vi "Variable Operation.vi"(8 "error in (no error)":errorcluster, 9 "Variable Tree":refnum<vi>, 10 "Variable Data":T1, 11 "Project in":refnum<class "Project.lvclass">) -> (0 "error out":errorcluster, 1 "Successful":bool, 3 "Project out":refnum<class "Project.lvclass">)   [LabVIEW 2015, in "Project.lvclass"]
uses:
  Project.lvclass
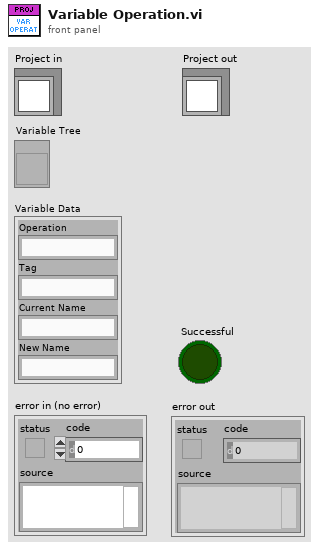
[diagram p1: front panel]
types:
  T1 = cluster{"Operation":string, "Tag":string, "Current Name":string, "New Name":string}
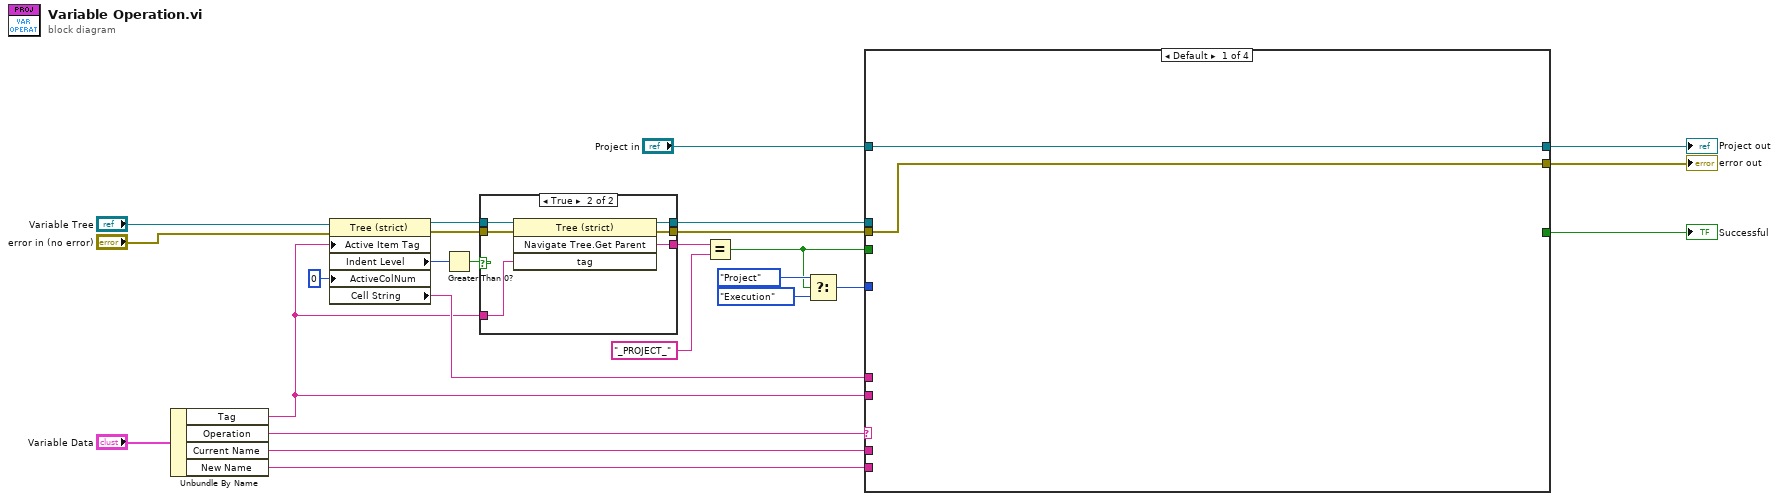
[diagram p0: block diagram]
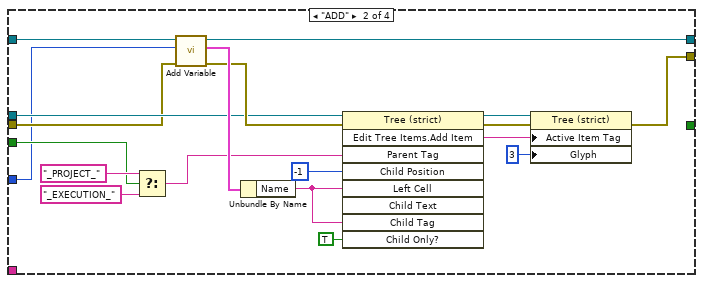
[diagram p2: hidden frame]
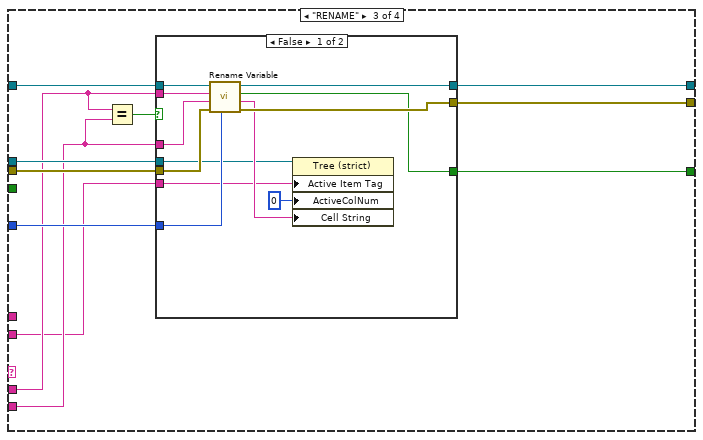
[diagram p3: hidden frame]
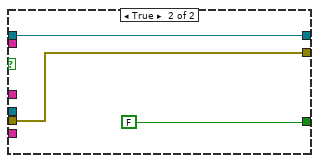
[diagram p4: hidden frame]
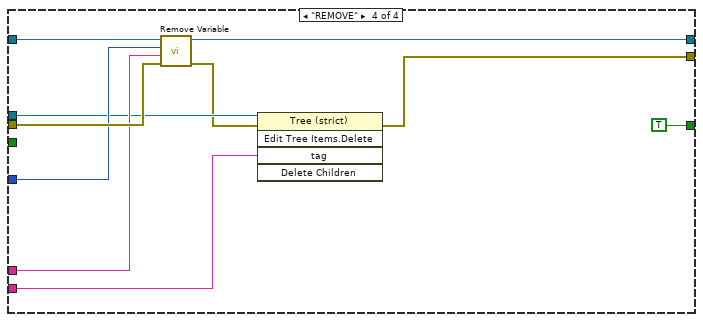
[diagram p5: hidden frame]
diagram:
  n1 = Unbundle By Name("Variable Data") -> ("Tag"=w4:string, "Operation"=w3:string, "Current Name"=w2:string, "New Name"=w1:string)
  n2 = property class="Tree (strict)"(reference="Variable Tree", error in="error in (no error)", "Active Item Tag"=w4, "ActiveColNum"=0 ("Active Cell:Active Column Number")) -> (reference out=w20:refnum<vi>, error out=w19:errorcluster, "Indent Level"=w15:i32, "Cell String"=w13:string)
  n3 = Greater Than 0?(x=w15) -> (x > 0?=w21:bool)
  n4 = case shown="True" w21 {
    tunnel: w4 -> [w28 w34]
    tunnel: w20 -> [w26 w33]
    tunnel: w19 -> [w27 w32]
    tunnel: [w28 w31] -> w18
    tunnel: [w26 w30] -> w17
    tunnel: [w27 w29] -> w16
    frame False {
    }
    frame True {
      n5 = invoke class="Tree (strict)" method="Navigate Tree.Get Parent"(reference=w33, error in=w32, "tag"=w34) -> (reference out=w30:refnum<vi>, error out=w29:errorcluster, "Navigate Tree:Get Parent"=w31:string)  [unwired: 1 in, 1 out]
    }
  }
  n6 = Equal?(x=w18, y="_PROJECT_") -> (x = y?=w9:bool)
  n7 = Select(t=enum16{"Project", "Execution"}."Project" ("Variable Type"), s=w9, f=enum16{"Project", "Execution"}."Execution" ("Variable Type")) -> (s? t:f=w8:enum16{"Project", "Execution"})
  n8 = case shown="Default" w3 {
    tunnel: "Project in" -> [w36 w55 w66 w91]
    tunnel: [w36 w51 w65 w90] -> w24
    tunnel: [w35 w45 w63 w83] -> w23
    tunnel: w17 -> [_ w43 w60 w86]
    tunnel: w9 -> [_ w39 _ _]
    tunnel: w16 -> [w35 w38 w64 w89]
    tunnel: w13 -> [_ _ _ w88]
    tunnel: [_ _ w62 TRUE ("Successful")] -> w12
    tunnel: w8 -> [_ w37 w59 w87]
    tunnel: w4 -> [_ _ w56 w84]
    tunnel: w2 -> [_ _ w58 _]
    tunnel: w1 -> [_ _ w57 _]
    frame Default {
    }
    frame "ADD" {
      n9 = Select(t="_PROJECT_", s=w39, f="_EXECUTION_" ("Child Tag")) -> (s? t:f=w40:string)
      n10 = call-dynamic "Add Variable.vi"("error in (no error)"=w38, "Variable Type"=w37, "Project in"=w55) -> ("error out"=w52:errorcluster, "Variable"=w54:cluster{"Name":string, "Value":variant}, "Project out"=w51:refnum<class "Project.lvclass">)  [unwired: 6 in]
      n11 = Unbundle By Name(w54) -> ("Name"=w53:string)
      n12 = invoke class="Tree (strict)" method="Edit Tree Items.Add Item"(reference=w43, error in=w52, "Parent Tag"=w40, "Child Position"=-1, "Left Cell"=w53, "Child Tag"=w53, "Child Only?"=TRUE) -> (reference out=w49:refnum<vi>, error out=w48:errorcluster, "Edit Tree Items:Add Item"=w47:string)  [unwired: 2 in, 6 out]
      n13 = property class="Tree (strict)"(reference=w49, error in=w48, "Active Item Tag"=w47, "Glyph"=3 ("Active Item:Symbol Index")) -> (error out=w45:errorcluster)  [unwired: 1 out]
    }
    frame "RENAME" {
      n14 = Equal?(x=w58, y=w57) -> (x = y?=w61:bool)
      n15 = case shown="False" w61 {
        tunnel: w66 -> [w78 w81]
        tunnel: [w77 w81] -> w65
        tunnel: w64 -> [w76 w80]
        tunnel: [w75 w80] -> w63
        tunnel: [w69 FALSE] -> w62
        tunnel: w58 -> [w74 _]
        tunnel: w57 -> [w73 _]
        tunnel: w60 -> [w68 _]
        tunnel: w59 -> [w72 _]
        tunnel: w56 -> [w67 _]
        frame False {
          n16 = call "Rename Variable.vi"("Variable Type"=w72, "error in (no error)"=w76, "New Name"=w73, "Current Name"=w74, "Project in"=w78) -> ("error out"=w75:errorcluster, "Name"=w70:string, "Successful"=w69:bool, "Project out"=w77:refnum<class "Project.lvclass">)  [unwired: 3 in]
          n17 = property class="Tree (strict)"(reference=w68, "Active Item Tag"=w67, "ActiveColNum"=0, "Cell String"=w70) -> ()  [unwired: 1 in, 2 out]
        }
        frame True {
        }
      }
    }
    frame "REMOVE" {
      n18 = call "Remove Variable.vi"("error in (no error)"=w89, "Name"=w88, "Variable Type"=w87, "Project in"=w91) -> ("error out"=w85:errorcluster, "Project out"=w90:refnum<class "Project.lvclass">)  [unwired: 6 in]
      n19 = invoke class="Tree (strict)" method="Edit Tree Items.Delete"(reference=w86, error in=w85, "tag"=w84) -> (error out=w83:errorcluster)  [unwired: 2 in, 4 out]
    }
  }
  "error out" <- w23
  "Project out" <- w24
  "Successful" <- w12
